vi "recordResultsToFile.vi"(8 "error in (no error)":errorcluster, 10 "Results":variant, 11 "ImageAnalyser in":refnum<class "ImageAnalyser.lvclass">) -> (0 "error out":errorcluster, 3 "ImageAnalyser out":refnum<class "ImageAnalyser.lvclass">)   [LabVIEW 2011, in "Tools.lvlib" / "Imaging.lvlib" / "ImageAnalyser.lvclass"]
uses:
  ImageAnalyser.lvclass
  Filing/FileNeologist/FileNeologist.lvclass
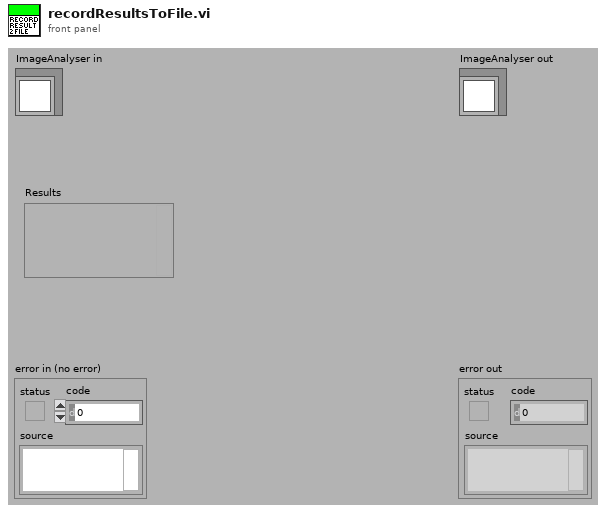
[diagram p1: front panel]
types:
  T1 = cluster{"Name":string, "Results":dbl[], "AnalysisType":string}
  T2 = enum16{"open", "replace", "create", "open or create", "replace or create", "replace or create with confirmation"}
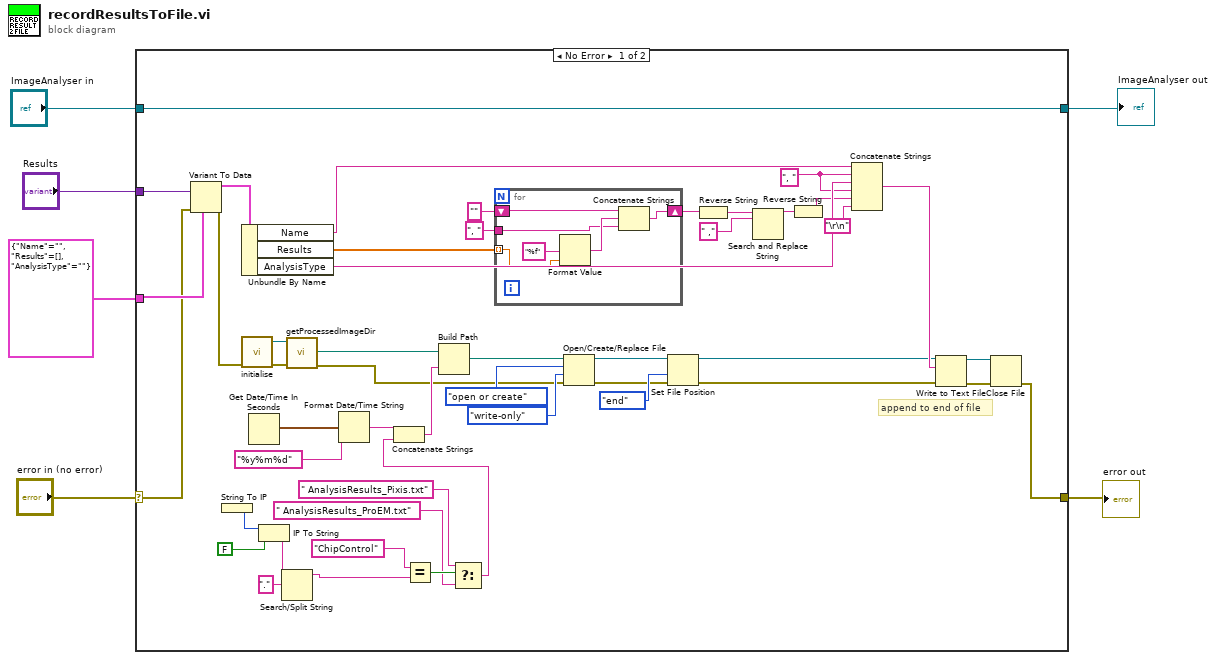
[diagram p0: block diagram]
diagram:
  n1 = case shown="No Error" "error in (no error)" {
    selector: "error in (no error)" -> [w50 w62]
    tunnel: [w21 w62] -> w5
    tunnel: [w54 w61] -> w3
    tunnel: "ImageAnalyser in" -> [w54 w61]
    tunnel: "Results" -> [w53 _]
    tunnel: T1 {"Name"="", "Results"=[], "AnalysisType"=""} ("output cluster") -> [w52 _]
    frame No Error {
      w32 = ", "
      # "append to end of file"
      n2 = Variant To Data(error in=w50, type=w52, Variant=w53) -> (data=w51:T1, error out=w47:errorcluster)
      n3 = String To IP() -> (0:w15:u32)  [unwired: 1 in]
      n4 = Unbundle By Name(w51) -> ("Name"=w35:string, "Results"=w41:dbl[], "AnalysisType"=w33:string)
      n5 = call "initialise.vi"("error in (no error)"=w47) -> ("error out"=w48:errorcluster, "FileNeologist out"=w49:refnum<class "FileNeologist.lvclass">)  [unwired: 9 in]
      n6 = Get Date/Time In Seconds() -> (seconds since 1Jan1904=w45:timestamp)
      n7 = IP To String(1:FALSE, 2:w15) -> (0:w14:string)
      n8 = Search/Split String(string=w14, search string/char (-)=".") -> (substring before match=w11:string)  [unwired: 1 in, 2 out]
      n9 = call-dynamic "getProcessedImageDir.vi"("error in (no error)"=w48, "FileNeologist in"=w49) -> ("error out"=w24:errorcluster, "Path"=w46:path)  [unwired: 7 in, 1 out]
      n10 = Format Date/Time String(time format string (%c)="%y%m%d", seconds (now)=w45) -> (date/time string=w43:string)  [unwired: 1 in]
      n11 = Equal?(x="ChipControl", y=w11) -> (x = y?=w10:bool)
      n12 = Select(t=" AnalysisResults_Pixis.txt", s=w10, f=" AnalysisResults_ProEM.txt") -> (s? t:f=w7:string)
      n13 = Concatenate Strings(w43, w7) -> (w42:string)
      n14 = Build Path(base path=w46, name or relative path=w42) -> (appended path=w28:path)
      n15 = for {
        tunnel: w41 -> [w59] mode=indexing
        shift-right: [w56] -> w39
        shift-left: "" -> [w58]
        tunnel: ", " -> [w55]
        n16 = Format Value(format string="%f", value (0)=w59) -> (output string=w57:string)  [unwired: 1 in]
        n17 = Concatenate Strings(w58, w57, w55) -> (w56:string)
      }
      n18 = Open/Create/Replace File(file path (use dialog)=w28, error in=w24, operation (0:open)=T2."open or create", access (0:read/write)=enum16{"read/write", "read-only", "write-only"}."write-only") -> (refnum out=w27:refnum<file>, error out=w18:errorcluster)  [unwired: 2 in, 1 out]
      n19 = Set File Position(refnum=w27, from (0:start)=enum16{"start", "end", "current"}."end", error in=w18) -> (refnum out=w20:refnum<file>, error out=w17:errorcluster)  [unwired: 1 in]
      n20 = Reverse String(1:w39) -> (0:w38:string)
      n21 = Search and Replace String(input string=w38, search string=" ,") -> (result string=w36:string)  [unwired: 6 in, 3 out]
      n22 = Reverse String(1:w36) -> (0:w31:string)
      n23 = Concatenate Strings(w35, w32, w33, w32, w31, "\r\n") -> (w29:string)
      n24 = Write to Text File(file (use dialog)=w20, text=w29, error in=w17) -> (refnum out=w22:refnum<file>, error out=w23:errorcluster)  [unwired: 1 in, 1 out]
      n25 = Close File(refnum=w22, error in=w23) -> (error out=w21:errorcluster)  [unwired: 1 out]
    }
    frame Error {
    }
  }
  "error out" <- w5
  "ImageAnalyser out" <- w3
